vi "Log Error to the Caller.vi"(8 "error in (no error)":errorcluster, 9 "Error to log":errorcluster, 11 "CO2 Actor in":refnum<class "CO2 Actor.lvclass">) -> (0 "error out":errorcluster, 3 "CO2 Actor out":refnum<class "CO2 Actor.lvclass">)   [LabVIEW 2015, in "cRIO-Carbondioxide.lvlib" / "CO2-Actor.lvlib" / "CO2 Actor.lvclass"]
uses:
  CO2 Actor.lvclass
  CO2 Actor.lvclass/CO2 Actor.ctl
  cRIO-CO2 Messages/Log Error Msg/Log Error Msg.lvclass/Log Error Msg.ctl
  <vilib>/ActorFramework/Message Enqueuer/Message Enqueuer.lvclass/Message Enqueuer.ctl
  <vilib>/ActorFramework/Message Enqueuer/Enqueue.vi
  <vilib>/ActorFramework/Message Priority Queue/Priority Enqueue.vi
  cRIO-CO2 Messages/Log Error Msg/Log Error Msg.lvclass
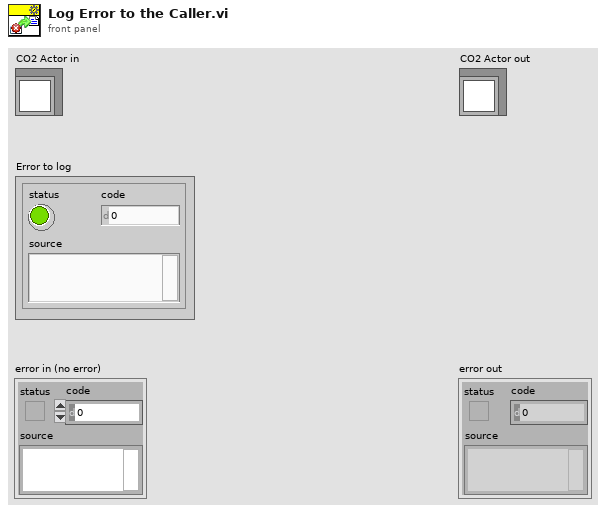
[diagram p1: front panel]
types:
  T1 = cluster{"status":bool, "code":bool, "source":bool}
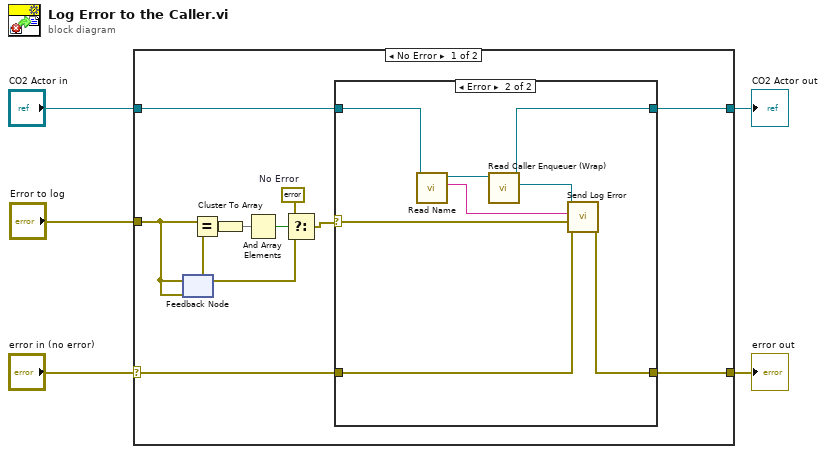
[diagram p0: block diagram]
diagram:
  n1 = case shown="No Error" "error in (no error)" {
    selector: "error in (no error)" -> [w16 w28]
    tunnel: [w13 w28] -> w4
    tunnel: [w15 w27] -> w2
    tunnel: "CO2 Actor in" -> [w14 w27]
    tunnel: "Error to log" -> [w7 _]
    frame No Error {
      w8 = errorcluster {"status"=FALSE, "code"=0, "source"=""}  # No Error
      n2 = feedback-in #1(w7) -> ()
      n3 = feedback #1(w7) -> (w9:errorcluster)
      n4 = Equal?(x=w7, y=w9) -> (x = y?=w12:T1)
      n5 = Cluster To Array(cluster=w12) -> (array=w11:bool[])
      n6 = And Array Elements(Boolean array=w11) -> (logical AND=w10:bool)
      n7 = Select(t=w8, s=w10, f=w9) -> (s? t:f=w6:errorcluster)
      n8 = case shown="Error" w6 {
        selector: w6 -> [_ w25]
        tunnel: w16 -> [w17 w20]
        tunnel: [w18 w24] -> w15
        tunnel: w14 -> [w18 w23]
        tunnel: [w17 w19] -> w13
        frame No Error {
        }
        frame Error {
          n9 = call "Read Name.vi"("CO2 Actor in"=w23) -> ("Name"=w21:string, "CO2 Actor out"=w22:refnum<class "CO2 Actor.lvclass">)  [unwired: 9 in]
          n10 = call "Read Caller Enqueuer (Wrap).vi"("CO2 Actor in"=w22) -> ("Actor Framework:Message Enqueuer"=w26:refnum<class "Message Enqueuer.lvclass">, "CO2 Actor out"=w24:refnum<class "CO2 Actor.lvclass">)  [unwired: 9 in]
          n11 = call "Send Log Error.vi"("error in (no error)"=w20, "error to log (no error)"=w25, "Source Name"=w21, "Message Enqueuer"=w26) -> ("error out"=w19:errorcluster)  [unwired: 6 in, 1 out]
        }
      }
    }
    frame Error {
    }
  }
  "error out" <- w4
  "CO2 Actor out" <- w2
